vi "Assert.vi"(6 "error code (1)":i32=1, 7 "Name":string, 8 "error in (no error)":errorcluster, 9 "ArtificialHierarchy":string[](array[string]), 10 "Assert?":bool, 11 "Assert in":refnum<class "Assert.lvclass">) -> (0 "error out":errorcluster, 3 "Assert out":refnum<class "Assert.lvclass">)   [LabVIEW 2009, in "Caraya.lvlib" / "Assert.lvclass"]
doc: "Defines how assertion should be handled. Default implementation renders an error if assertion fails."
uses:
  Assert.lvclass
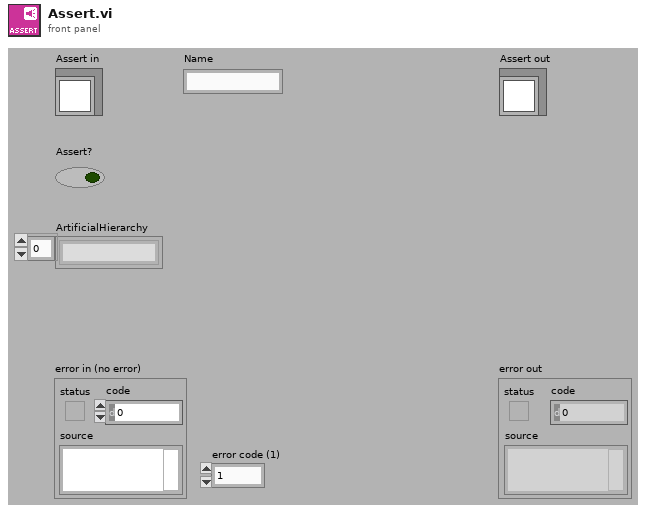
[diagram p1: front panel]
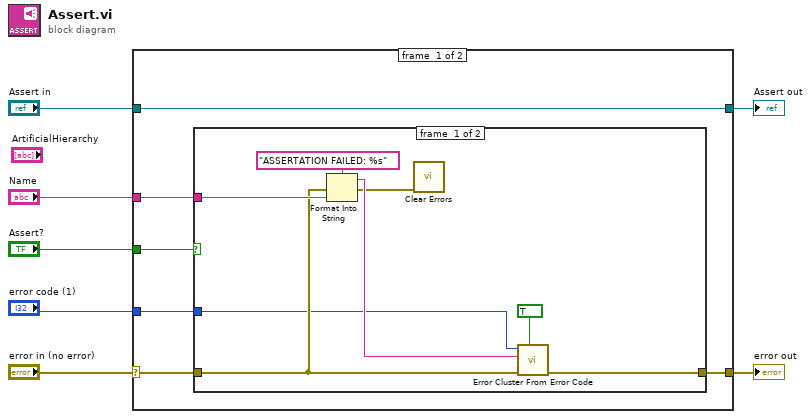
[diagram p0: block diagram]
diagram:
  n1 = case shown="No Error" "error in (no error)" {
    selector: "error in (no error)" -> [w11 w24]
    tunnel: [w10 w24] -> w6
    tunnel: [w13 w23] -> w4
    tunnel: "Assert in" -> [w13 w23]
    tunnel: "Assert?" -> [w12 _]
    tunnel: "Name" -> [w9 _]
    tunnel: "error code (1)" -> [w8 _]
    frame #0 {
      n2 = case shown="False" w12 {
        tunnel: w11 -> [w18 w22]
        tunnel: [w21 w22] -> w10
        tunnel: w9 -> [w19 _]
        tunnel: w8 -> [w14 _]
        frame #0 {
          n3 = Format Into String(format string="ASSERTATION FAILED: %s", error in=w18, w19) -> (resulting string=w17:string, error out=w16:errorcluster)  [unwired: 1 in]
          n4 = call <vilib>:"Clear Errors.vi"("error in (no error)"=w16) -> ()  [unwired: 6 in, 1 out]
          n5 = call <vilib>:"Error Cluster From Error Code.vi"("show call chain? (False)"=TRUE, "error in (no error)"=w18, "error message (\"\")"=w17, "error code (0)"=w14) -> ("error out"=w21:errorcluster)  [unwired: 5 in]
        }
        frame #1 {
        }
      }
    }
    frame #1 {
    }
  }
  "error out" <- w6
  "Assert out" <- w4
